vi "TCP Listener Stop.vi"(8 "error in (no error)":errorcluster, 10 "Listener Error":errorcluster, 11 "tWorkerController in":refnum<class "tWorkerController.lvclass">) -> (0 "error out":errorcluster, 3 "tWorkerController out":refnum<class "tWorkerController.lvclass">)   [LabVIEW 2013, in "tWorkerController.lvlib" / "tWorkerController.lvclass"]
doc: "Allows unexpected errors from the listener to be handled. An expected error is generated when this actor is stopped, but if this happens this command will be queued after the stop command and will eventually get dropped on the floor, which is what we want."
uses:
  tWorkerController.lvclass
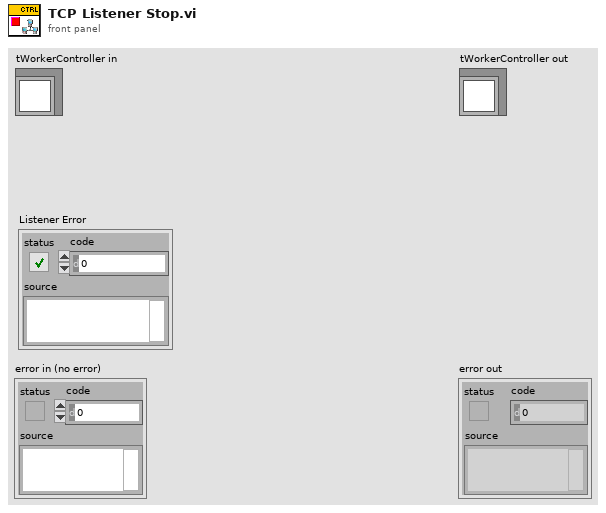
[diagram p1: front panel]
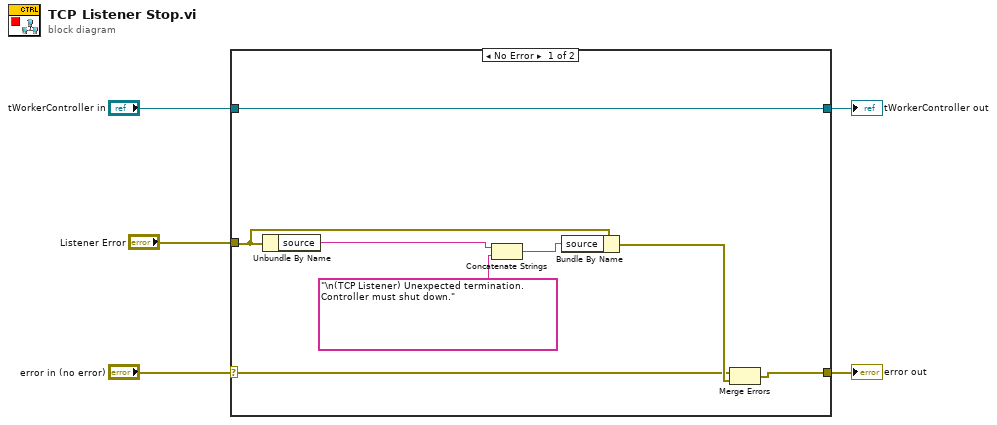
[diagram p0: block diagram]
diagram:
  n1 = case shown="No Error" "error in (no error)" {
    selector: "error in (no error)" -> [w6 w15]
    tunnel: [w7 w15] -> w4
    tunnel: [w11 w14] -> w2
    tunnel: "tWorkerController in" -> [w11 w14]
    tunnel: "Listener Error" -> [w10 _]
    frame No Error {
      n2 = Unbundle By Name(w10) -> ("source"=w13:string)
      n3 = Concatenate Strings(w13, "\n(TCP Listener) Unexpected termination.  Controller must shut down." ("string")) -> (w9:string)
      n4 = Bundle By Name(cluster=w10, "source"=w9) -> (w8:errorcluster)
      n5 = Merge Errors(w6, w8) -> (w7:errorcluster)
    }
    frame Error {
    }
  }
  "error out" <- w4
  "tWorkerController out" <- w2
